vi "Shooter Target Speed.vi"() -> ()   [LabVIEW 2019]
panel:
  in  "Long Shot RPM?":bool
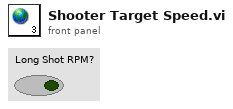
[diagram p1: front panel]
diagram:
